vi "Global.vi"() -> ()   [LabVIEW 2012]
panel:
  in  "String":string
  out "Waveform Chart":dbl(graph)
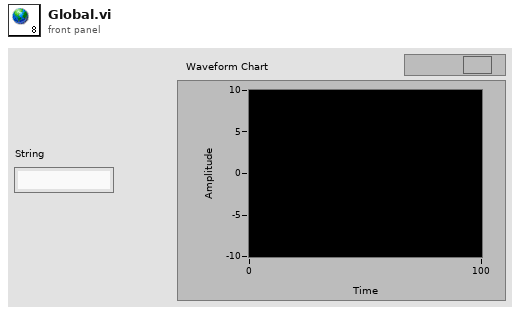
[diagram p1: front panel]
diagram:
